vi "DefaultSettings.vi"(3 "Defaults":cluster{"name":string, "Content":string}[](array[cluster])=[{"name"="1 flat (200-7000)_filter.txt", "Content"="200.000000\t7000.000000\n"}, {"name"="2 JC vln 4 band  (200-780-1740-2930-7000)_filter.txt", "Content"="200.000000\t780.000000\t1740.000000\t2930.000000\t7000.000000\n"}, {"name"="24_colors.txt", "Content"="\u0000æ\u0019K\u0000<´K\u0000ÿá\u0019\u0000\u0000È\u0000õ0\u0000\u0014´\u0000Fðð\u0000ð2æ\u0000Òõ<\u0000ú¾¾\u0000\u0000\u0000æ¾ÿ\u0000ªn(\u0000ÿúÈ\u0000\u0000\u0000\u0000ªÿÃ\u0000\u0000\u0000ÿ×´\u0000\u0000\u0000\u0000\u0000\u0000\u0000\u0000\u0000zÿ\u0000\u0000ù\u0000\u0000°\"g"}, {"name"="3 JC vln 5 band (200-780-1740-3000-5200-7000)_filter.txt", "Content"="200.000000\t780.000000\t1740.000000\t3000.000000\t5200.000000\t7000.000000\n"}, {"name"="4 JC vla 4 band {200-650-1500-2700-6300}_filter.txt", "Content"="200.000000\t650.000000\t1575.000000\t2450.000000\t6300.000000\n"}, {"name"="Bark  (200-300-400-510-630-770-920-1080-1270-1480-1700-2000-2330-3000-3150-3700-4400-5300-6400-7700-9500)_filter.txt", "Content"="200.000000\t300.000000\t400.000000\t510.000000\t630.000000\t770.000000\t920.000000\t1080.000000\t1270.000000\t1480.000000\t1720.000000\t2000.000000\t2320.000000\t2700.000000\t3150.000000\t3700.000000\t4400.000000\t5300.000000\t6400.000000\t7700.000000\t9500.000000\n"}, {"name"="Default_calib.txt", "Content"="Voltage=<1.000000E+0/>\nMicrophone=<1.000000E+0/>\nAccelerometer=<1.000000E+0/>\nVibrometer=<1.000000E+0/>\nHammer=<1.000000E+0/>\nPiezo=<1.000000E+0/>\nFlip=<0.000000E+0/>\n"}, {"name"="DefaultColors.txt", "Content"="\u0000\u0000Üh\u0000Yïÿ\u0000ÿ\u0000\u0000\u0000•»•\u0000ÿ\u0000\u0000\u0000+++\u0000\u001d\u0000ÿ\u0000*ÿT"}, {"name"="DefaultNotes.txt", "Content"="Instrument info: \n\n\n\nTemplate: \n\nMeasured at: \n\nMic: Behringer EDM 8000\n\nMic distance: 20 cm\n\nSoundcard: Mackie, Onxy Producer2.2 \n \n"}, {"name"="HV 24 Obie Rig_template.txt", "Content"="Name of test=<Asdfsdfa--Asdfsdfa 01/>\nDate=<3862638541/>\nLocation=<Home/>\nTemplate=<1 1 HV 24 Obie Rig/>\nSoundcard=<Line (Onyx Producer 2-2)/>\nresolution=<24/>\nSampling rate=<48000/>\nCh1 Gain =<20.000000/>\nCh2 Gain=<20.000000/>\nSample time (s)=<0.300000/>\nPre-trigger (s)=<0.001000/>\nHammer Threshold=<0.010000/>\nPositions=<12/>\nTaps/Position=<5/>\nSet Names=<H,V/>\nFreq resolution=<1.000000/>\nHammer cutoff=<0.025000/>\nMic cutoff=<0.250000/>\nDouble bounce =<1.000000/>\nHammer Cal=<1.000000/>\ndB Offset=<0.000000/>\nAccel Cal=<1.000000/>\nVibrometer Cal=<1.000000/>\nMic Cal=<1.000000/>\nOutput=<2/>\nVoltage Cal=<1.000000/>\nVibrometer Port=<ASRL27::INSTR/>\nRange=<50/>\nHigh Pass=<2/>\nBandwidth=<25/>\nX Range=<2.000000E+2\t1.000000E+4\t1.000000E+1\t1.000000E+2\t2.000000E+2\n0.000000E+0\t5.000000E-2\t2.500000E-2\t2.500000E-3\t0.000000E+0\n0.000000E+0\t3.000000E-1\t1.000000E-1\t1.000000E-2\t0.000000E+0\n2.000000E+2\t1.000000E+4\t1.000000E+1\t1.000000E+2\t1.000000E+3\n/>\nY Range=<-2.500000E+1\t0.000000E+0\t5.000000E+0\t1.000000E+0\t-2.500000E+1\n-1.000000E-1\t1.000000E+0\t2.500000E-1\t5.000000E-2\t0.000000E+0\n-1.000000E+0\t1.000000E+0\t5.000000E-1\t1.000000E-1\t-1.000000E+0\n-1.100000E+1\t2.900000E+1\t2.000000E+0\t5.000000E-1\t-1.000000E+1\n/>\ndB Spread=<40.000000/>\nTrigger=<0/>\nCh_1=<2/>\nCh_2=<1/>\nflip?=<false/>\n60Hz=<false/>\nTime offset=<0.000000/>\nPiezo Cal=<1.000000/>\nDefault Notes=<Instrument info: \n\n\n \nTemplate: HV 24  Obie 26\n\nMeasured at: \n\nMic: Behringer ECM 8000 at 20 cm\nSoundcard:  Mackie Onyx Producer 2.2 \n/>\nTom=<false/>\n"}, {"name"="JC 5_colors.txt", "Content"="\u0000\u0000\u0000\u0000\u0000È\u0006\u0000\u0000\u0000†ÿ\u0000o´\u0000\u0000yBÿ"}, {"name"="Scratchpad Obie 26_template.txt", "Content"="Name of test=<1 1 Scratchpad Obie 26/>\nDate=<3862644811/>\nLocation=<Scratch/>\nTemplate=<1 1 Scratchpad Obie 26/>\nSoundcard=<Line (Onyx Producer 2-2)/>\nresolution=<24/>\nSampling rate=<48000/>\nCh1 Gain =<0.000000/>\nCh2 Gain=<0.000000/>\nSample time (s)=<0.300000/>\nPre-trigger (s)=<0.001000/>\nHammer Threshold=<0.011083/>\nPositions=<1/>\nTaps/Position=<10/>\nSet Names=<H/>\nFreq resolution=<1.000000/>\nHammer cutoff=<0.018750/>\nMic cutoff=<0.300000/>\nDouble bounce =<1.000000/>\nHammer Cal=<1.000000/>\ndB Offset=<0.000000/>\nAccel Cal=<1.000000/>\nVibrometer Cal=<1.000000/>\nMic Cal=<1.000000/>\nOutput=<2/>\nVoltage Cal=<1.000000/>\nVibrometer Port=<ASRL27::INSTR/>\nRange=<20/>\nHigh Pass=<2/>\nBandwidth=<25/>\nX Range=<2.000000E+2\t1.000000E+4\t1.000000E+1\t1.000000E+2\t2.000000E+2\n-1.000000E-2\t5.000000E-2\t2.000000E-2\t2.000000E-3\t0.000000E+0\n-1.000000E-1\t4.000000E-1\t1.000000E-1\t2.000000E-2\t-1.000000E-1\n2.000000E+2\t7.000000E+3\t1.000000E+1\t1.000000E+2\t1.000000E+3\n/>\nY Range=<-2.500000E+1\t0.000000E+0\t2.500000E+1\t1.000000E+0\t-2.500000E+1\n-2.000000E-2\t1.000000E+0\t2.000000E-1\t5.000000E-2\t0.000000E+0\n-1.000000E+0\t1.000000E+0\t5.000000E-1\t1.000000E-1\t-1.000000E+0\n-1.300000E+1\t2.200000E+1\t2.500000E+0\t5.000000E-1\t-1.250000E+1\n/>\ndB Spread=<35.000000/>\nTrigger=<0/>\nCh_1=<2/>\nCh_2=<1/>\nflip?=<false/>\n60Hz=<false/>\nTime offset=<0.000000/>\nPiezo Cal=<1.000000/>\nDefault Notes=<Instrument info: \n\n\nMic:  Behringer ECM 8000 mic at 20 cm.\nMic distance: 20 cm. \nHammer: Obie 26 Thor />\nTom=<false/>\n"}, {"name"="ScratchPad_template.txt", "Content"="Name of test=<ScratchPad/>\nDate=<0/>\nLocation=<Home/>\nDefault Template=<ScratchPad/>\nSoundcard=<1-2 (OCTA-CAPTURE)/>\nresolution=<32/>\nSampling rate=<48000/>\nCh1 Gain =<10.000000/>\nCh2 Gain=<20.000000/>\nSample time (s)=<0.300000/>\nPre-trigger (s)=<0.001000/>\nHammer Threshold=<0.010000/>\nPositions=<1/>\nTaps/Position=<5/>\nSet Names=<H/>\nFreq resolution=<1.000000/>\nHammer cutoff=<0.025000/>\nMic cutoff=<0.250000/>\nDouble bounce =<0.010000/>\nHammer Cal=<1.000000/>\ndB Offset=<0.000000/>\nAccel Cal=<1.000000/>\nVibrometer Cal=<1.000000/>\nMic Cal=<49.380000/>\nOutput=<2/>\nVoltage Cal=<13.800000/>\nVibrometer Port=<ASRL27::INSTR/>\nRange=<4/>\nHigh Pass=<2/>\nBandwidth=<4/>\nX Range=<2.000000E+2\t1.000000E+4\t2.500000E+3\t5.000000E+2\t2.000000E+2\n0.000000E+0\t5.000000E-2\t2.500000E-2\t2.500000E-3\t0.000000E+0\n0.000000E+0\t3.000000E-1\t1.000000E-1\t1.000000E-2\t0.000000E+0\n2.000000E+2\t1.000000E+4\t1.000000E+1\t1.000000E+2\t2.000000E+2\n/>\nY Range=<-2.500000E+1\t0.000000E+0\t5.000000E+0\t1.000000E+0\t-2.500000E+1\n-1.000000E-1\t1.000000E+0\t2.500000E-1\t5.000000E-2\t-1.000000E-1\n-1.000000E+0\t1.000000E+0\t5.000000E-1\t1.000000E-1\t-1.000000E+0\n-3.000000E+1\t3.000000E+1\t5.000000E+0\t1.000000E+0\t-3.000000E+1\n/>\ndB Spread=<40.000000/>\nTrigger=<0/>\nCh_1=<1/>\nCh_2=<2/>\n"}, {"name"="TagFilters.txt", "Content"="{\"Pattern (eg. H,V)\":\"hv\",\"File type\":{\"AvR\":true,\"AvC\":false,\"trf\":true,\"wav\":false,\"All\":false},\"keywords 1\":\"2001.10\",\"keywords 2\":\"\",\"keywords 3\":\"\"}"}], 6 "error in (no error)":errorcluster, 9 "Task":enum16{"Load to VI", "Save to Disk"}(ring), 11 "path (use dialog)":path=path "/Users/crogers/Documents/LabVIEW Data/ViolinCompare") -> (1 "No Errors?":bool)   [LabVIEW 2022 SP3]
panel:
  out "Array":T1(array[cluster])=[{{"name"="A Octaves_filter.txt", "Content"="440.000000\t880.000000\t1760.000000\t3520.000000\t7040.000000\n"}, "error out"={"status"=FALSE, "code"=0, "source"=""}}, {{"name"="Acoustic Test_template.txt", "Content"="Name of test=<Acoustic Test/>\nDate=<3622387832/>\nLocation=<Home/>\nDefault Template=<Acoustic Test/>\nSoundcard=<OCTA-CAPTURE/>\nresolution=<32/>\nSampling rate=<48000/>\nCh1 Gain =<15.000000/>\nCh2 Gain=<20.000000/>\nSample time (s)=<0.300000/>\nPre-trigger (s)=<0.001000/>\nHammer Threshold=<0.077459/>\nPositions=<1/>\nTaps/Position=<5/>\nSet Names=<H/>\nFreq resolution=<1.000000/>\nHammer cutoff=<0.109860/>\nMic cutoff=<0.097861/>\nDouble bounce =<0.010000/>\nHammer Cal=<1.000000/>\ndB Offset=<0.000000/>\nAccel Cal=<1.000000/>\nVibrometer Cal=<20.000000/>\nMic Cal=<49.380000/>\nOutput=<2/>\nVoltage Cal=<13.400000/>\nVibrometer Port=<ASRL27::INSTR/>\nRange=<4/>\nHigh Pass=<2/>\nBandwidth=<4/>\nX Range=<2.000000E+2\t1.000000E+4\t1.000000E+1\t1.000000E+2\t2.000000E+2\n5.291005E-4\t3.000000E-1\t2.000000E-1\t1.000000E-2\t2.000000E-1\n0.000000E+0\t3.000000E-1\t1.000000E-1\t1.000000E-2\t0.000000E+0\n2.000000E+2\t1.000000E+4\t1.000000E+1\t1.000000E+2\t1.000000E+3\n/>\nY Range=<-2.500000E+1\t0.000000E+0\t5.000000E+0\t1.000000E+0\t-2.500000E+1\n-1.000000E-2\t1.000000E-1\t2.000000E-2\t5.000000E-3\t0.000000E+0\n-1.000000E-1\t1.000000E-1\t5.000000E-2\t1.000000E-2\t-1.000000E-1\n-6.100000E+1\t-2.100000E+1\t2.000000E+0\t5.000000E-1\t-6.000000E+1\n/>\ndB Spread=<40.000000/>\nInput=<1/>\nCh_1=<2/>\nCh_2=<1/>\n"}, "error out"={"status"=FALSE, "code"=0, "source"=""}}, {{"name"="Bridge ScratchPad_template.txt", "Content"="Name of test=<Bridge ScratchPad/>\nDate=<3622387832/>\nLocation=<Home/>\nDefault Template=<Bridge ScratchPad/>\nSoundcard=<Built-in Microph/>\nresolution=<32/>\nSampling rate=<48000/>\nCh1 Gain =<15.000000/>\nCh2 Gain=<20.000000/>\nSample time (s)=<5.000000/>\nPre-trigger (s)=<1.000000/>\nHammer Threshold=<0.077459/>\nPositions=<1/>\nTaps/Position=<5/>\nSet Names=<H/>\nFreq resolution=<1.000000/>\nHammer cutoff=<5.000000/>\nMic cutoff=<5.000000/>\nDouble bounce =<0.010000/>\nHammer Cal=<1.000000/>\ndB Offset=<0.000000/>\nAccel Cal=<1.000000/>\nVibrometer Cal=<20.000000/>\nMic Cal=<49.380000/>\nOutput=<2/>\nVoltage Cal=<13.400000/>\nVibrometer Port=<ASRL27::INSTR/>\nRange=<4/>\nHigh Pass=<2/>\nBandwidth=<4/>\nX Range=<2.000000E+2\t1.000000E+4\t1.000000E+1\t1.000000E+2\t2.000000E+2\n0.000000E+0\t5.000000E+0\t1.000000E+0\t2.000000E-1\t0.000000E+0\n0.000000E+0\t5.000000E+0\t1.000000E+0\t2.000000E-1\t0.000000E+0\n2.000000E+2\t1.000000E+4\t1.000000E+1\t1.000000E+2\t1.000000E+3\n/>\nY Range=<-2.500000E+1\t0.000000E+0\t5.000000E+0\t1.000000E+0\t-2.500000E+1\n-1.000000E+0\t1.000000E+0\t5.000000E-1\t1.000000E-1\t-1.000000E+0\n-1.000000E+0\t1.000000E+0\t5.000000E-1\t1.000000E-1\t-1.000000E+0\n-6.100000E+1\t-2.100000E+1\t2.000000E+0\t5.000000E-1\t-6.000000E+1\n/>\ndB Spread=<40.000000/>\nInput=<1/>\nCh_1=<2/>\nCh_2=<1/>\n"}, "error out"={"status"=FALSE, "code"=0, "source"=""}}, {{"name"="Curtin Bands_filter.txt", "Content"="200.000000\t780.000000\t1740.000000\t2930.000000\t7000.000000\n"}, "error out"={"status"=FALSE, "code"=0, "source"=""}}, {{"name"="JC Admit H laser_template.txt", "Content"="Name of test=<JC Admit H laser/>\nDate=<3645005742/>\nLocation=<Home/>\nDefault Template=<JC Admit H/>\nSoundcard=<1-2 (OCTA-CAPTURE)/>\nresolution=<32/>\nSampling rate=<48000/>\nCh1 Gain =<5.000000/>\nCh2 Gain=<26.000000/>\nSample time (s)=<0.300000/>\nPre-trigger (s)=<0.001000/>\nHammer Threshold=<0.010000/>\nPositions=<1/>\nTaps/Position=<5/>\nSet Names=<H/>\nFreq resolution=<1.000000/>\nHammer cutoff=<0.025000/>\nMic cutoff=<0.250000/>\nDouble bounce =<0.010000/>\nHammer Cal=<23.600000/>\ndB Offset=<0.000000/>\nAccel Cal=<1.000000/>\nVibrometer Cal=<40.000000/>\nMic Cal=<66.000000/>\nOutput=<2/>\nVoltage Cal=<1.000000/>\nVibrometer Port=<ASRL27::INSTR/>\nRange=<4/>\nHigh Pass=<0/>\nBandwidth=<3/>\nX Range=<2.000000E+2\t1.000000E+4\t1.000000E+1\t1.000000E+2\t2.000000E+2\n0.000000E+0\t5.000000E-2\t2.500000E-2\t2.500000E-3\t0.000000E+0\n0.000000E+0\t3.000000E-1\t1.000000E-1\t1.000000E-2\t0.000000E+0\n2.000000E+2\t1.000000E+4\t1.000000E+1\t1.000000E+2\t1.000000E+3\n/>\nY Range=<-2.500000E+1\t0.000000E+0\t5.000000E+0\t1.000000E+0\t-2.500000E+1\n-1.000000E-1\t1.000000E-1\t5.000000E-2\t1.000000E-2\t-1.000000E-1\n-1.000000E-1\t1.000000E-1\t5.000000E-2\t1.000000E-2\t-1.000000E-1\n5.000000E+0\t4.500000E+1\t2.000000E+0\t5.000000E-1\t6.000000E+0\n/>\ndB Spread=<40.000000/>\nTrigger=<0/>\nCh_1=<1/>\nCh_2=<2/>\n"}, "error out"={"status"=FALSE, "code"=0, "source"=""}}, {{"name"="JC Admit.HV laser_template.txt", "Content"="Name of test=<JC Admit.HV laser/>\nDate=<0/>\nLocation=<Home/>\nDefault Template=<JC Admit.HV/>\nSoundcard=<3-4 (OCTA-CAPTURE)/>\nresolution=<32/>\nSampling rate=<48000/>\nCh1 Gain =<9.000000/>\nCh2 Gain=<29.000000/>\nSample time (s)=<0.300000/>\nPre-trigger (s)=<0.001000/>\nHammer Threshold=<0.010000/>\nPositions=<1/>\nTaps/Position=<5/>\nSet Names=<H,T,V/>\nFreq resolution=<1.000000/>\nHammer cutoff=<0.025000/>\nMic cutoff=<0.250000/>\nDouble bounce =<0.010000/>\nHammer Cal=<23.600000/>\ndB Offset=<0.000000/>\nAccel Cal=<1.000000/>\nVibrometer Cal=<40.000000/>\nMic Cal=<66.000000/>\nOutput=<3/>\nVoltage Cal=<1.000000/>\nVibrometer Port=<ASRL27::INSTR/>\nRange=<4/>\nHigh Pass=<2/>\nBandwidth=<4/>\nX Range=<2.000000E+2\t1.000000E+4\t2.500000E+3\t5.000000E+2\t2.500000E+3\n0.000000E+0\t5.000000E-2\t2.500000E-2\t2.500000E-3\t0.000000E+0\n0.000000E+0\t3.000000E-1\t1.000000E-1\t1.000000E-2\t0.000000E+0\n2.000000E+2\t1.000000E+4\t1.000000E+1\t1.000000E+2\t1.000000E+3\n/>\nY Range=<-2.500000E+1\t0.000000E+0\t5.000000E+0\t1.000000E+0\t-2.500000E+1\n-1.000000E-1\t1.000000E-1\t5.000000E-2\t1.000000E-2\t-1.000000E-1\n-1.000000E-1\t1.000000E-1\t5.000000E-2\t1.000000E-2\t-1.000000E-1\n-3.000000E+1\t3.000000E+1\t5.000000E+0\t1.000000E+0\t-3.000000E+1\n/>\ndB Spread=<40.000000/>\nTrigger=<0/>\nCh_1=<1/>\nCh_2=<2/>\n"}, "error out"={"status"=FALSE, "code"=0, "source"=""}}, {{"name"="JC H 12 radiation_template.txt", "Content"="Name of test=<JC H 12 radiation/>\nDate=<3647857419/>\nLocation=<Home/>\nDefault Template=<H 12 radiation/>\nSoundcard=<1-2 (OCTA-CAPTURE)/>\nresolution=<32/>\nSampling rate=<48000/>\nCh1 Gain =<10.000000/>\nCh2 Gain=<20.500000/>\nSample time (s)=<0.300000/>\nPre-trigger (s)=<0.001000/>\nHammer Threshold=<0.010000/>\nPositions=<12/>\nTaps/Position=<5/>\nSet Names=<H/>\nFreq resolution=<1.000000/>\nHammer cutoff=<0.025000/>\nMic cutoff=<0.250000/>\nDouble bounce =<0.010000/>\nHammer Cal=<23.600000/>\ndB Offset=<0.000000/>\nAccel Cal=<1.000000/>\nVibrometer Cal=<40.000000/>\nMic Cal=<66.000000/>\nOutput=<3/>\nVoltage Cal=<1.000000/>\nVibrometer Port=<ASRL27::INSTR/>\nRange=<4/>\nHigh Pass=<0/>\nBandwidth=<3/>\nX Range=<2.000000E+2\t1.000000E+4\t1.000000E+1\t1.000000E+2\t2.000000E+2\n0.000000E+0\t5.000000E-2\t2.500000E-2\t2.500000E-3\t0.000000E+0\n-2.000000E-2\t3.000000E-1\t1.000000E-1\t1.000000E-2\t0.000000E+0\n1.500000E+2\t1.000000E+4\t1.000000E+1\t1.000000E+2\t1.000000E+3\n/>\nY Range=<-2.500000E+1\t0.000000E+0\t5.000000E+0\t1.000000E+0\t-2.500000E+1\n-1.000000E-1\t1.000000E+0\t2.500000E-1\t5.000000E-2\t0.000000E+0\n-1.000000E+0\t1.000000E+0\t5.000000E-1\t1.000000E-1\t-1.000000E+0\n-1.000000E+1\t3.000000E+1\t2.000000E+0\t5.000000E-1\t-1.000000E+1\n/>\ndB Spread=<30.000000/>\nTrigger=<0/>\nCh_1=<1/>\nCh_2=<2/>\n"}, "error out"={"status"=FALSE, "code"=0, "source"=""}}, {{"name"="JC H 7 radiation_template.txt", "Content"="Name of test=<JC H 7 radiation/>\nDate=<3647859161/>\nLocation=<Home/>\nDefault Template=<JC H 7 radiation/>\nSoundcard=<1-2 (OCTA-CAPTURE)/>\nresolution=<32/>\nSampling rate=<48000/>\nCh1 Gain =<5.000000/>\nCh2 Gain=<20.500000/>\nSample time (s)=<0.300000/>\nPre-trigger (s)=<0.001000/>\nHammer Threshold=<0.010000/>\nPositions=<7/>\nTaps/Position=<5/>\nSet Names=<H/>\nFreq resolution=<1.000000/>\nHammer cutoff=<0.025000/>\nMic cutoff=<0.250000/>\nDouble bounce =<0.010000/>\nHammer Cal=<23.600000/>\ndB Offset=<0.000000/>\nAccel Cal=<1.000000/>\nVibrometer Cal=<40.000000/>\nMic Cal=<66.000000/>\nOutput=<2/>\nVoltage Cal=<1.000000/>\nVibrometer Port=<ASRL27::INSTR/>\nRange=<4/>\nHigh Pass=<0/>\nBandwidth=<3/>\nX Range=<2.000000E+2\t1.000000E+4\t1.000000E+1\t1.000000E+2\t2.000000E+2\n0.000000E+0\t5.000000E-2\t2.500000E-2\t2.500000E-3\t0.000000E+0\n-2.000000E-2\t3.000000E-1\t1.000000E-1\t1.000000E-2\t0.000000E+0\n1.500000E+2\t1.000000E+4\t1.000000E+1\t1.000000E+2\t1.000000E+3\n/>\nY Range=<-2.500000E+1\t0.000000E+0\t5.000000E+0\t1.000000E+0\t-2.500000E+1\n-1.000000E-1\t1.000000E+0\t2.500000E-1\t5.000000E-2\t0.000000E+0\n-1.000000E+0\t1.000000E+0\t5.000000E-1\t1.000000E-1\t-1.000000E+0\n-1.000000E+1\t3.000000E+1\t2.000000E+0\t5.000000E-1\t-1.000000E+1\n/>\ndB Spread=<30.000000/>\nTrigger=<0/>\nCh_1=<1/>\nCh_2=<2/>\n"}, "error out"={"status"=FALSE, "code"=0, "source"=""}}, {{"name"="JC HV 24 radiation_template.txt", "Content"="Name of test=<JC HV 24 radiation/>\nDate=<3648550918/>\nLocation=<Home/>\nDefault Template=<JCS HV 24/>\nSoundcard=<1-2 (OCTA-CAPTURE)/>\nresolution=<32/>\nSampling rate=<48000/>\nCh1 Gain =<5.000000/>\nCh2 Gain=<20.500000/>\nSample time (s)=<0.300000/>\nPre-trigger (s)=<0.001000/>\nHammer Threshold=<0.010000/>\nPositions=<12/>\nTaps/Position=<5/>\nSet Names=<H,V/>\nFreq resolution=<1.000000/>\nHammer cutoff=<0.025000/>\nMic cutoff=<0.250000/>\nDouble bounce =<0.010000/>\nHammer Cal=<23.600000/>\ndB Offset=<0.000000/>\nAccel Cal=<1.000000/>\nVibrometer Cal=<40.000000/>\nMic Cal=<66.000000/>\nOutput=<2/>\nVoltage Cal=<1.000000/>\nVibrometer Port=<ASRL27::INSTR/>\nRange=<4/>\nHigh Pass=<0/>\nBandwidth=<3/>\nX Range=<2.000000E+2\t1.000000E+4\t1.000000E+1\t1.000000E+2\t2.000000E+2\n0.000000E+0\t5.000000E-2\t2.500000E-2\t2.500000E-3\t0.000000E+0\n0.000000E+0\t3.000000E-1\t1.000000E-1\t1.000000E-2\t0.000000E+0\n2.000000E+2\t1.000000E+4\t1.000000E+1\t1.000000E+2\t1.000000E+3\n/>\nY Range=<-2.500000E+1\t0.000000E+0\t5.000000E+0\t1.000000E+0\t-2.500000E+1\n-1.000000E-1\t1.000000E-1\t5.000000E-2\t1.000000E-2\t-1.000000E-1\n-1.000000E-1\t1.000000E-1\t5.000000E-2\t1.000000E-2\t-1.000000E-1\n-3.000000E+0\t2.700000E+1\t2.000000E+0\t5.000000E-1\t-2.000000E+0\n/>\ndB Spread=<30.000000/>\nTrigger=<0/>\nCh_1=<1/>\nCh_2=<2/>\n"}, "error out"={"status"=FALSE, "code"=0, "source"=""}}, {{"name"="JC violin 200-7000 Flat_filter.txt", "Content"="200.000000\t7000.000000\n"}, "error out"={"status"=FALSE, "code"=0, "source"=""}}, {{"name"="JC violin 200-780-1740-2930-7000_filter.txt", "Content"="200.000000\t780.000000\t1740.000000\t2930.000000\t7000.000000\n"}, "error out"={"status"=FALSE, "code"=0, "source"=""}}, {{"name"="JC violin 200-780-7000_filter.txt", "Content"="200.000000\t780.000000\t7000.000000\n"}, "error out"={"status"=FALSE, "code"=0, "source"=""}}, {{"name"="Laser Admitance ScratchPad_template.txt", "Content"="Name of test=<Laser Admitance ScratchPad/>\nDate=<0/>\nLocation=<Home/>\nDefault Template=<Scratch Admittance/>\nSoundcard=<1-2 (OCTA-CAPTURE)/>\nresolution=<32/>\nSampling rate=<48000/>\nCh1 Gain =<10.000000/>\nCh2 Gain=<20.500000/>\nSample time (s)=<0.300000/>\nPre-trigger (s)=<0.001000/>\nHammer Threshold=<0.010000/>\nPositions=<5/>\nTaps/Position=<1/>\nSet Names=<H/>\nFreq resolution=<1.000000/>\nHammer cutoff=<0.025000/>\nMic cutoff=<0.250000/>\nDouble bounce =<0.010000/>\nHammer Cal=<23.600000/>\ndB Offset=<0.000000/>\nAccel Cal=<1.000000/>\nVibrometer Cal=<40.000000/>\nMic Cal=<66.000000/>\nOutput=<3/>\nVoltage Cal=<1.000000/>\nVibrometer Port=<ASRL27::INSTR/>\nRange=<5/>\nHigh Pass=<1/>\nBandwidth=<3/>\nX Range=<2.000000E+2\t1.000000E+4\t2.500000E+3\t5.000000E+2\t2.500000E+3\n0.000000E+0\t5.000000E-2\t2.500000E-2\t2.500000E-3\t0.000000E+0\n0.000000E+0\t3.000000E-1\t1.000000E-1\t1.000000E-2\t0.000000E+0\n2.000000E+2\t1.000000E+4\t1.000000E+1\t1.000000E+2\t1.000000E+3\n/>\nY Range=<-2.500000E+1\t0.000000E+0\t5.000000E+0\t1.000000E+0\t-2.500000E+1\n-1.000000E-1\t1.000000E-1\t5.000000E-2\t1.000000E-2\t-1.000000E-1\n-1.000000E-1\t1.000000E-1\t5.000000E-2\t1.000000E-2\t-1.000000E-1\n-3.000000E+1\t3.000000E+1\t5.000000E+0\t1.000000E+0\t-3.000000E+1\n/>\ndB Spread=<40.000000/>\nInput=<0/>\nCh_1=<1/>\nCh_2=<2/>\n"}, "error out"={"status"=FALSE, "code"=0, "source"=""}}, {{"name"="ObieAlto 200-650-1500-2700-6300_filter.txt", "Content"="200.000000\t650.000000\t1575.000000\t2450.000000\t6300.000000\n"}, "error out"={"status"=FALSE, "code"=0, "source"=""}}, {{"name"="Old_ScratchPad_template.txt", "Content"="Name of test=<Old_ScratchPad/>\nDate=<3622387832/>\nLocation=<Home/>\nDefault Template=<ScratchPad/>\nSoundcard=<Built-in Microph/>\nresolution=<32/>\nSampling rate=<48000/>\nCh1 Gain =<15.000000/>\nCh2 Gain=<20.000000/>\nSample time (s)=<0.300000/>\nPre-trigger (s)=<0.001000/>\nHammer Threshold=<0.050000/>\nPositions=<1/>\nTaps/Position=<5/>\nSet Names=<H/>\nFreq resolution=<1.000000/>\nHammer cutoff=<0.030000/>\nMic cutoff=<0.100000/>\nDouble bounce =<0.010000/>\nHammer Cal=<1.000000/>\ndB Offset=<0.000000/>\nAccel Cal=<1.000000/>\nVibrometer Cal=<20.000000/>\nMic Cal=<49.380000/>\nOutput=<2/>\nVoltage Cal=<13.400000/>\nVibrometer Port=<ASRL27::INSTR/>\nRange=<4/>\nHigh Pass=<2/>\nBandwidth=<4/>\nX Range=<2.000000E+2\t1.000000E+4\t1.000000E+1\t1.000000E+2\t2.000000E+2\n0.000000E+0\t5.000000E-2\t2.500000E-2\t2.500000E-3\t0.000000E+0\n0.000000E+0\t3.000000E-1\t1.000000E-1\t1.000000E-2\t0.000000E+0\n2.000000E+2\t1.000000E+4\t1.000000E+1\t1.000000E+2\t1.000000E+3\n/>\nY Range=<-2.500000E+1\t0.000000E+0\t5.000000E+0\t1.000000E+0\t-2.500000E+1\n-1.000000E-2\t1.000000E-1\t2.000000E-2\t5.000000E-3\t0.000000E+0\n-1.000000E-1\t1.000000E-1\t5.000000E-2\t1.000000E-2\t-1.000000E-1\n-6.100000E+1\t-2.100000E+1\t2.000000E+0\t5.000000E-1\t-6.000000E+1\n/>\ndB Spread=<40.000000/>\nInput=<0/>\nCh_1=<2/>\nCh_2=<1/>\n"}, "error out"={"status"=FALSE, "code"=0, "source"=""}}, {{"name"="Radiation ScratchPad_template.txt", "Content"="Name of test=<Radiation ScratchPad/>\nDate=<0/>\nLocation=<Home/>\nDefault Template=<JC Scratch Radiation/>\nSoundcard=<1-2 (OCTA-CAPTURE)/>\nresolution=<32/>\nSampling rate=<48000/>\nCh1 Gain =<10.000000/>\nCh2 Gain=<20.500000/>\nSample time (s)=<0.300000/>\nPre-trigger (s)=<0.001000/>\nHammer Threshold=<0.010000/>\nPositions=<1/>\nTaps/Position=<5/>\nSet Names=<H/>\nFreq resolution=<1.000000/>\nHammer cutoff=<0.025000/>\nMic cutoff=<0.250000/>\nDouble bounce =<0.010000/>\nHammer Cal=<23.600000/>\ndB Offset=<0.000000/>\nAccel Cal=<1.000000/>\nVibrometer Cal=<40.000000/>\nMic Cal=<66.000000/>\nOutput=<2/>\nVoltage Cal=<1.000000/>\nVibrometer Port=<ASRL27::INSTR/>\nRange=<4/>\nHigh Pass=<2/>\nBandwidth=<4/>\nX Range=<2.000000E+2\t1.000000E+4\t2.500000E+3\t5.000000E+2\t2.500000E+3\n0.000000E+0\t5.000000E-2\t2.500000E-2\t2.500000E-3\t0.000000E+0\n0.000000E+0\t3.000000E-1\t1.000000E-1\t1.000000E-2\t0.000000E+0\n2.000000E+2\t1.000000E+4\t1.000000E+1\t1.000000E+2\t1.000000E+3\n/>\nY Range=<-2.500000E+1\t0.000000E+0\t5.000000E+0\t1.000000E+0\t-2.500000E+1\n-1.000000E-1\t1.000000E-1\t5.000000E-2\t1.000000E-2\t-1.000000E-1\n-1.000000E-1\t1.000000E-1\t5.000000E-2\t1.000000E-2\t-1.000000E-1\n-3.000000E+1\t3.000000E+1\t5.000000E+0\t1.000000E+0\t-3.000000E+1\n/>\ndB Spread=<40.000000/>\nTrigger=<0/>\nCh_1=<1/>\nCh_2=<2/>\n"}, "error out"={"status"=FALSE, "code"=0, "source"=""}}, {{"name"="ScratchPad_template.txt", "Content"="Name of test=<ScratchPad/>\nDate=<0/>\nLocation=<Home/>\nDefault Template=<ScratchPad/>\nSoundcard=<1-2 (OCTA-CAPTURE)/>\nresolution=<32/>\nSampling rate=<48000/>\nCh1 Gain =<10.000000/>\nCh2 Gain=<20.000000/>\nSample time (s)=<0.300000/>\nPre-trigger (s)=<0.001000/>\nHammer Threshold=<0.010000/>\nPositions=<1/>\nTaps/Position=<5/>\nSet Names=<H/>\nFreq resolution=<1.000000/>\nHammer cutoff=<0.025000/>\nMic cutoff=<0.250000/>\nDouble bounce =<0.010000/>\nHammer Cal=<1.000000/>\ndB Offset=<0.000000/>\nAccel Cal=<1.000000/>\nVibrometer Cal=<1.000000/>\nMic Cal=<49.380000/>\nOutput=<2/>\nVoltage Cal=<13.800000/>\nVibrometer Port=<ASRL27::INSTR/>\nRange=<4/>\nHigh Pass=<2/>\nBandwidth=<4/>\nX Range=<2.000000E+2\t1.000000E+4\t2.500000E+3\t5.000000E+2\t2.500000E+3\n0.000000E+0\t5.000000E-2\t2.500000E-2\t2.500000E-3\t0.000000E+0\n0.000000E+0\t3.000000E-1\t1.000000E-1\t1.000000E-2\t0.000000E+0\n2.000000E+2\t1.000000E+4\t1.000000E+1\t1.000000E+2\t1.000000E+3\n/>\nY Range=<-2.500000E+1\t0.000000E+0\t5.000000E+0\t1.000000E+0\t-2.500000E+1\n-1.000000E-1\t1.000000E-1\t5.000000E-2\t1.000000E-2\t-1.000000E-1\n-1.000000E-1\t1.000000E-1\t5.000000E-2\t1.000000E-2\t-1.000000E-1\n-3.000000E+1\t3.000000E+1\t5.000000E+0\t1.000000E+0\t-3.000000E+1\n/>\ndB Spread=<40.000000/>\nTrigger=<0/>\nCh_1=<1/>\nCh_2=<2/>\n"}, "error out"={"status"=FALSE, "code"=0, "source"=""}}, {{"name"="TapTones ScratchPad_template.txt", "Content"="Name of test=<TapTones ScratchPad/>\nDate=<3622387832/>\nLocation=<Home/>\nDefault Template=<TapTones ScratchPad/>\nSoundcard=<Built-in Microph/>\nresolution=<32/>\nSampling rate=<48000/>\nCh1 Gain =<15.000000/>\nCh2 Gain=<20.000000/>\nSample time (s)=<1.000000/>\nPre-trigger (s)=<0.500000/>\nHammer Threshold=<0.100000/>\nPositions=<1/>\nTaps/Position=<5/>\nSet Names=<H/>\nFreq resolution=<1.000000/>\nHammer cutoff=<1.000000/>\nMic cutoff=<1.000000/>\nDouble bounce =<0.100000/>\nHammer Cal=<1.000000/>\ndB Offset=<0.000000/>\nAccel Cal=<1.000000/>\nVibrometer Cal=<20.000000/>\nMic Cal=<49.380000/>\nOutput=<2/>\nVoltage Cal=<13.400000/>\nVibrometer Port=<ASRL27::INSTR/>\nRange=<4/>\nHigh Pass=<2/>\nBandwidth=<4/>\nX Range=<2.000000E+2\t1.000000E+4\t1.000000E+1\t1.000000E+2\t2.000000E+2\n0.000000E+0\t5.000000E+0\t1.000000E+0\t2.000000E-1\t0.000000E+0\n0.000000E+0\t5.000000E+0\t1.000000E+0\t2.000000E-1\t0.000000E+0\n2.000000E+2\t1.000000E+4\t1.000000E+1\t1.000000E+2\t1.000000E+3\n/>\nY Range=<-2.500000E+1\t0.000000E+0\t5.000000E+0\t1.000000E+0\t-2.500000E+1\n-1.000000E+0\t1.000000E+0\t5.000000E-1\t1.000000E-1\t-1.000000E+0\n-1.000000E+0\t1.000000E+0\t5.000000E-1\t1.000000E-1\t-1.000000E+0\n1.240000E+2\t1.640000E+2\t2.000000E+0\t5.000000E-1\t1.240000E+2\n/>\ndB Spread=<60.000000/>\nTrigger=<1/>\nCh_1=<2/>\nCh_2=<1/>\n"}, "error out"={"status"=FALSE, "code"=0, "source"=""}}]
  # "You should run this to grab all the files from the\nDetault Settings and put them in the array below so that\nwhen people run and do not have a Violin Compare folder\nthey will get it pre-poulated with these."
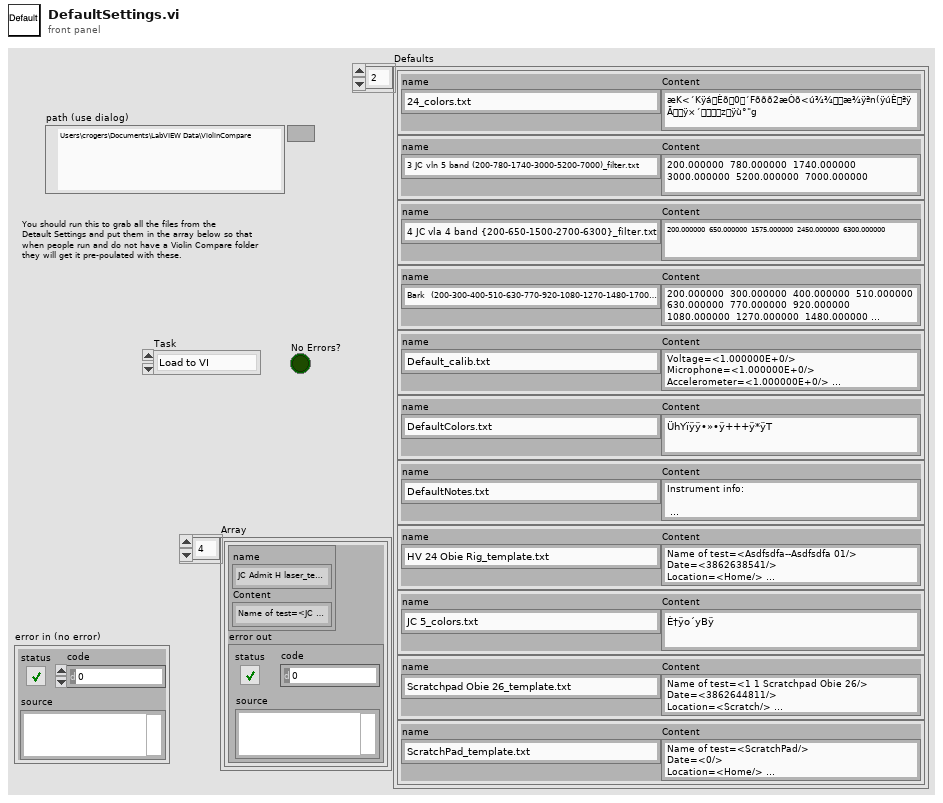
[diagram p1: front panel]
types:
  T1 = cluster{cluster{"name":string, "Content":string}, "error out":errorcluster}[]
  T2 = cluster{cluster{"name":string, "Content":string}, "error out":errorcluster}
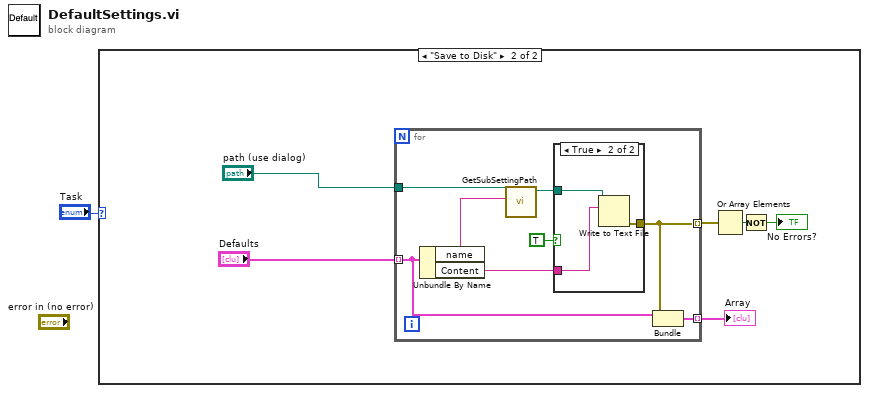
[diagram p0: block diagram]
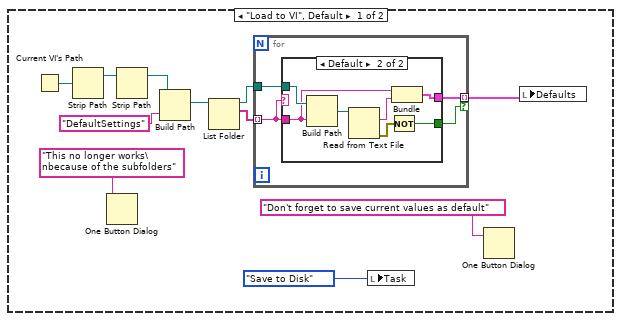
[diagram p2: hidden frame]
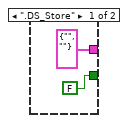
[diagram p3: hidden frame]
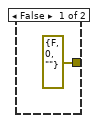
[diagram p4: hidden frame]
diagram:
  n1 = case shown="\"Save to Disk\"" "Task" {
    frame "Load to VI", Default {
      n2 = Current VI's Path() -> (path=w12:path)
      n3 = Strip Path(path=w12) -> (stripped path=w11:path)  [unwired: 1 out]
      n4 = One Button Dialog(message="This no longer works\nbecause of the subfolders") -> ()  [unwired: 1 in, 1 out]
      n5 = Strip Path(path=w11) -> (stripped path=w9:path)  [unwired: 1 out]
      n6 = Build Path(base path=w9, name or relative path="DefaultSettings") -> (appended path=w6:path)
      n7 = List Folder(path=w6) -> (path out=w7:path, filenames=w8:string[])  [unwired: 3 in, 2 out]
      n8 = for {
        tunnel: w8 -> [w13] mode=indexing
        tunnel: w7 -> [w16]
        tunnel: [w15] -> w5 mode=indexing if=w14
        n9 = case shown="Default" w13 {
          tunnel: w16 -> [_ w25]
          tunnel: w13 -> [_ w22]
          tunnel: [cluster{string, string} {"", ""} w21] -> w15
          tunnel: [FALSE w19] -> w14
          frame ".DS_Store" {
          }
          frame Default {
            n10 = Build Path(base path=w25, name or relative path=w22) -> (appended path=w24:path)
            n11 = Read from Text File(file (use dialog)=w24) -> (text=w23:string, error out=w20:errorcluster)  [unwired: 3 in, 2 out]
            n12 = Not(x=w20) -> (.not. x?=w19:bool)
            n13 = Bundle(w22, w23) -> (w21:cluster{string, string})  [unwired: 1 in]
          }
        }
      }
      n14 = local write "Task"(enum16{"Load to VI", "Save to Disk"}."Save to Disk" ("Task")) -> ()
      n15 = One Button Dialog(message="Don't forget to save current values as default") -> ()  [unwired: 1 in, 1 out]
      n16 = local write "Defaults"(w5) -> ()
    }
    frame "Save to Disk" {
      n17 = for {
        tunnel: "path (use dialog)" -> [w35]
        tunnel: "Defaults" -> [w38] mode=indexing
        tunnel: [w37] -> w30 mode=indexing
        tunnel: [w36] -> w28 mode=indexing
        n18 = Unbundle By Name(w38) -> ("name"=w34:string, "Content"=w39:string)
        n19 = call "GetSubSettingPath.vi"("settings file name"=w34, "LabVIEW Data Path"=w35) -> ("settings file path"=w33:path)  [unwired: 8 in, 1 out]
        n20 = case shown="True" TRUE {
          tunnel: w39 -> [_ w43]
          tunnel: [errorcluster {"status"=FALSE, "code"=0, "source"=""} ("error out") w42] -> w37
          tunnel: w33 -> [_ w41]
          frame False {
          }
          frame True {
            n21 = Write to Text File(file (use dialog)=w41, text=w43) -> (error out=w42:errorcluster)  [unwired: 2 in, 2 out]
          }
        }
        n22 = Bundle(w38, "error out"=w37) -> (w36:T2)  [unwired: 1 in]
      }
      "Array" <- w28
      n23 = Or Array Elements(Boolean array=w30) -> (logical OR=w29:bool)
      n24 = Not(x=w29) -> (.not. x?=→"No Errors?":bool)
    }
  }
